vi "cache tag indices.vi"(8 "error in":errorcluster, 9 "index cluster":variant, 10 "channel classification":T1, 11 "RT Resource Usage runtime in":refnum<class "RT Resource Usage runtime.lvclass">) -> (0 "error out":errorcluster, 3 "RT Resource Usage runtime out":refnum<class "RT Resource Usage runtime.lvclass">)   [LabVIEW 2017, in "RT Resource Usage runtime.lvclass"]
uses:
  RT Resource Usage runtime.lvclass
  <vilib>/NI/Tag Bus Module Framework/channel/channel classification.ctl
  configuration/input data indices.ctl
  RT Resource Usage runtime.lvclass/RT Resource Usage runtime.ctl
  configuration/output data indices.ctl
  configuration/parameter data indices.ctl
  configuration/result data indices.ctl
  configuration/RT Resource Usage configuration.lvclass
  <vilib>/NI/Tag Bus Module Framework/channel/TBM channel.lvclass
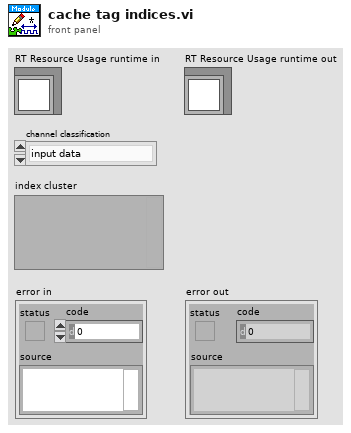
[diagram p1: front panel]
types:
  T1 = typedef "TBM channel.lvclass/channel classification.ctl" = enum16{"input data", "output data", "processing parameter", "processing result"}
  T2 = typedef "RT Resource Usage configuration.lvclass/input data indices.ctl" = cluster{"Array of Double.CPU_Usage":i32, "Double.Mean_CPU_Usage":i32, "Double.FreePhyMemory":i32, "Double.FreePhyMemoryPercent":i32, "Double.FreeVirtualMemory":i32, "Double.FreeVirtualMemoryPercent":i32, "Double.PrimaryDiskFree":i32, "Double.PrimaryDiskFreePercent":i32}
  T3 = typedef "RT Resource Usage configuration.lvclass/output data indices.ctl" = cluster{"fmwk_placeholder":i32}
  T4 = typedef "RT Resource Usage configuration.lvclass/parameter data indices.ctl" = cluster{"fmwk_placeholder":i32}
  T5 = typedef "RT Resource Usage configuration.lvclass/result data indices.ctl" = cluster{"fmwk_placeholder":i32}
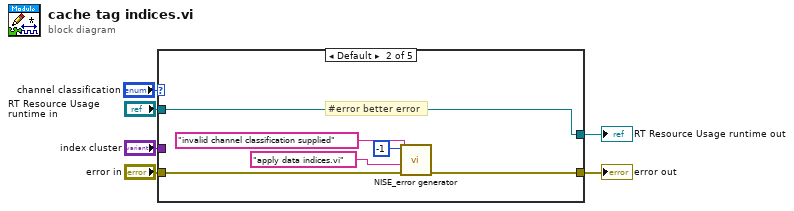
[diagram p0: block diagram]
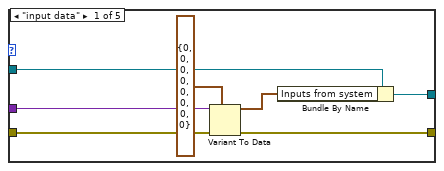
[diagram p2: hidden frame]
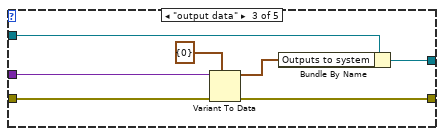
[diagram p3: hidden frame]
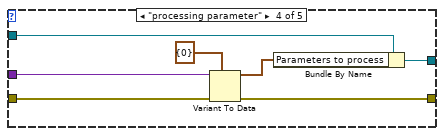
[diagram p4: hidden frame]
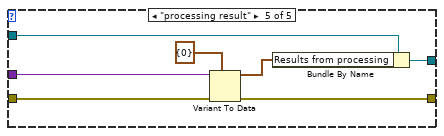
[diagram p5: hidden frame]
diagram:
  n1 = case shown="Default" "channel classification" {
    tunnel: "error in" -> [w11 w18 w24 w31 w38]
    tunnel: [w9 w17 w22 w29 w36] -> w5
    tunnel: [w12 w19 w25 w32 w39] -> w4
    tunnel: "RT Resource Usage runtime in" -> [w13 w19 w26 w33 w40]
    tunnel: "index cluster" -> [w10 _ w23 w30 w37]
    frame "input data" {
      n2 = Variant To Data(error in=w11, type=T2 {"Array of Double.CPU_Usage"=0, "Double.Mean_CPU_Usage"=0, "Double.FreePhyMemory"=0, "Double.FreePhyMemoryPercent"=0, "Double.FreeVirtualMemory"=0, "Double.FreeVirtualMemoryPercent"=0, "Double.PrimaryDiskFree"=0, "Double.PrimaryDiskFreePercent"=0} ("Cluster"), Variant=w10) -> (data=w8:T2, error out=w9:errorcluster)
      n3 = Bundle By Name(cluster=w13, "Inputs from system"=w8) -> (w12:refnum<class "RT Resource Usage runtime.lvclass">)
    }
    frame Default {
      # "#error better error"
      n4 = call <vilib>:"NISE_error generator.vi"("error in"=w18, "source"="apply data indices.vi", "append error message"="invalid channel classification supplied", "error code (0)"=-1) -> ("error out"=w17:errorcluster)  [unwired: 5 in]
    }
    frame "output data" {
      n5 = Variant To Data(error in=w24, type=T3 {"fmwk_placeholder"=0} ("Cluster"), Variant=w23) -> (data=w21:T3, error out=w22:errorcluster)
      n6 = Bundle By Name(cluster=w26, "Outputs to system"=w21) -> (w25:refnum<class "RT Resource Usage runtime.lvclass">)
    }
    frame "processing parameter" {
      n7 = Variant To Data(error in=w31, type=T4 {"fmwk_placeholder"=0} ("Cluster"), Variant=w30) -> (data=w28:T4, error out=w29:errorcluster)
      n8 = Bundle By Name(cluster=w33, "Parameters to process"=w28) -> (w32:refnum<class "RT Resource Usage runtime.lvclass">)
    }
    frame "processing result" {
      n9 = Variant To Data(error in=w38, type=T5 {"fmwk_placeholder"=0} ("Cluster"), Variant=w37) -> (data=w35:T5, error out=w36:errorcluster)
      n10 = Bundle By Name(cluster=w40, "Results from processing"=w35) -> (w39:refnum<class "RT Resource Usage runtime.lvclass">)
    }
  }
  "error out" <- w5
  "RT Resource Usage runtime out" <- w4
